vi "Conf EZ.vi"(0 "VISA Resource Name":refnum<visa-resource-name>, 1 "Voltage/Freq/Period Conf":T2={"Range (5:Auto)"=enum."Auto", "Resolution (5:Default)"=enum."Default"}, 2 "Current Conf":T4={"Range (3:Auto)"=enum."Auto", "Resolution (3:Least)"=enum."Least"}, 3 "Resistance Conf":T3={"Range (7:Auto)"=enum."Auto", "Resolution (5:Default)"=enum."Default"}, 5 "Channel List(empty)":string, 7 "Set/Check (F:Set)":bool, 9 "Measurement (1:DC Volt)":T5(ring)=enum."DC Voltage", 11 "error in (no error)":errorcluster, 12 "Temperature Conf":T1={"Transducer Type (0:TC)"=enum."Thermocouple", "Thermocouple Type (8:Last)"=enum."Default (Last)", "Thermistor Type (3: Last)"=enum."Default (Last)", "RTD Type (2:Last)"=enum."Default (Last)"}, 13 "Digital (0:Byte)":u16(ring) items=["Byte"], 14 "Totalizer (0:Read)":enum16{"Read", "Read and Reset"}(ring)) -> (4 "VISA Resource Name Out":refnum<visa-resource-name>, 8 "Configuration?":string, 15 "error out":errorcluster)   [LabVIEW 2018, in "Agilent 34970.lvlib"]
doc: "This VI lets you configure the instrument for simple voltage, current, resistance, temperature, freq/period and, digital/totalizer measurements as well as setting up the scan list. Looking at the block diagram of \"HP34970A Advanced Scan Example.vi\", this VI replaces the specific measurment configuration commands (e.g. Conf Voltage) as well as the Conf Scan List VI. The trigger and read VIs are still needed to take a measurement. For more information on the different ways to take a measurment, refer to the context help and block diagram of the \"HP34970A Advanced Scan Example.vi\".\n\n* Note * There was a bug in the old driver giving the option to read a word from the digital port. This is not possible with the CONF command. To read a word, according to the documentation, put both digital input channels in the same scan list. The readings will be taken simultaneously and given the same timestamp."
uses:
  Agilent 34970.lvlib
panel:
  out "Command":string
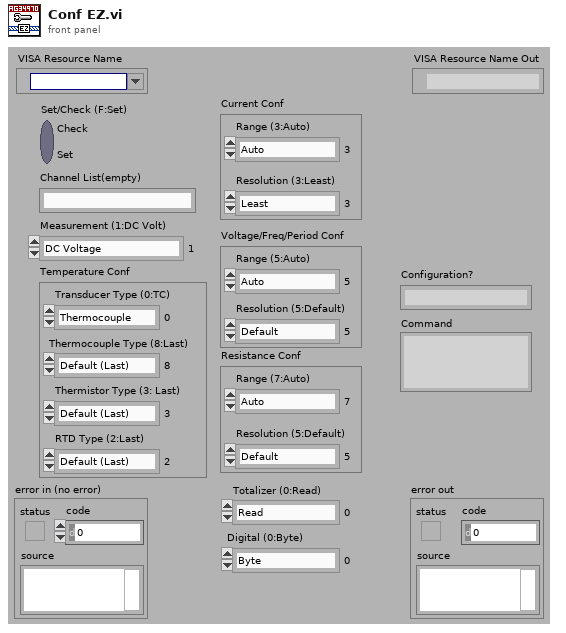
[diagram p1: front panel]
types:
  T1 = cluster{"Transducer Type (0:TC)":enum16{"Thermocouple", "Thermistor", "RTD", "4-Wire RTD", "Default (Last)"}, "Thermocouple Type (8:Last)":enum16{"B", "E", "J", "K", "N", "R", "S", "T", "Default (Last)"}, "Thermistor Type (3: Last)":enum16{"2252", "5000", "10000", "Default (Last)"}, "RTD Type (2:Last)":enum16{"85", "91", "Default (Last)"}}
  T2 = cluster{"Range (5:Auto)":enum16{"100 mV", "1 V", "10 V", "100 V", "300 V", "Auto", "Minimum", "Maximum"}, "Resolution (5:Default)":enum16{"4 1/2", "5 1/2", "6 1/2", "Least", "Highest", "Default"}}
  T3 = cluster{"Range (7:Auto)":enum16{"100 Ohm", "1 kOhm", "10 kOhm", "100 kOhm", "1 MOhm", "10 MOhm", "100 MOhm", "Auto", "Minimum", "Maximum"}, "Resolution (5:Default)":enum16{"4 1/2", "5 1/2", "6 1/2", "Least", "Highest", "Default"}}
  T4 = cluster{"Range (3:Auto)":enum16{"10 mA", "100 mA", "1 A", "Auto", "Minimum", "Maximum"}, "Resolution (3:Least)":enum16{"4 1/2", "5 1/2", "6 1/2", "Least", "Highest", "Default"}}
  T5 = enum16{"Temperature", "DC Voltage", "AC Voltage", "DC Current", "AC Current", "Resistance", "4-Wire Resistance", "Frequency", "Period", "Digital", "Totalizer"}
  T6 = enum16{"Thermocouple", "Thermistor", "RTD", "4-Wire RTD", "Default (Last)"}
  T7 = enum16{"B", "E", "J", "K", "N", "R", "S", "T", "Default (Last)"}
  T8 = enum16{"2252", "5000", "10000", "Default (Last)"}
  T9 = enum16{"100 mV", "1 V", "10 V", "100 V", "300 V", "Auto", "Minimum", "Maximum"}
  T10 = enum16{"4 1/2", "5 1/2", "6 1/2", "Least", "Highest", "Default"}
  T11 = enum16{"100 Ohm", "1 kOhm", "10 kOhm", "100 kOhm", "1 MOhm", "10 MOhm", "100 MOhm", "Auto", "Minimum", "Maximum"}
  T12 = enum16{"10 mA", "100 mA", "1 A", "Auto", "Minimum", "Maximum"}
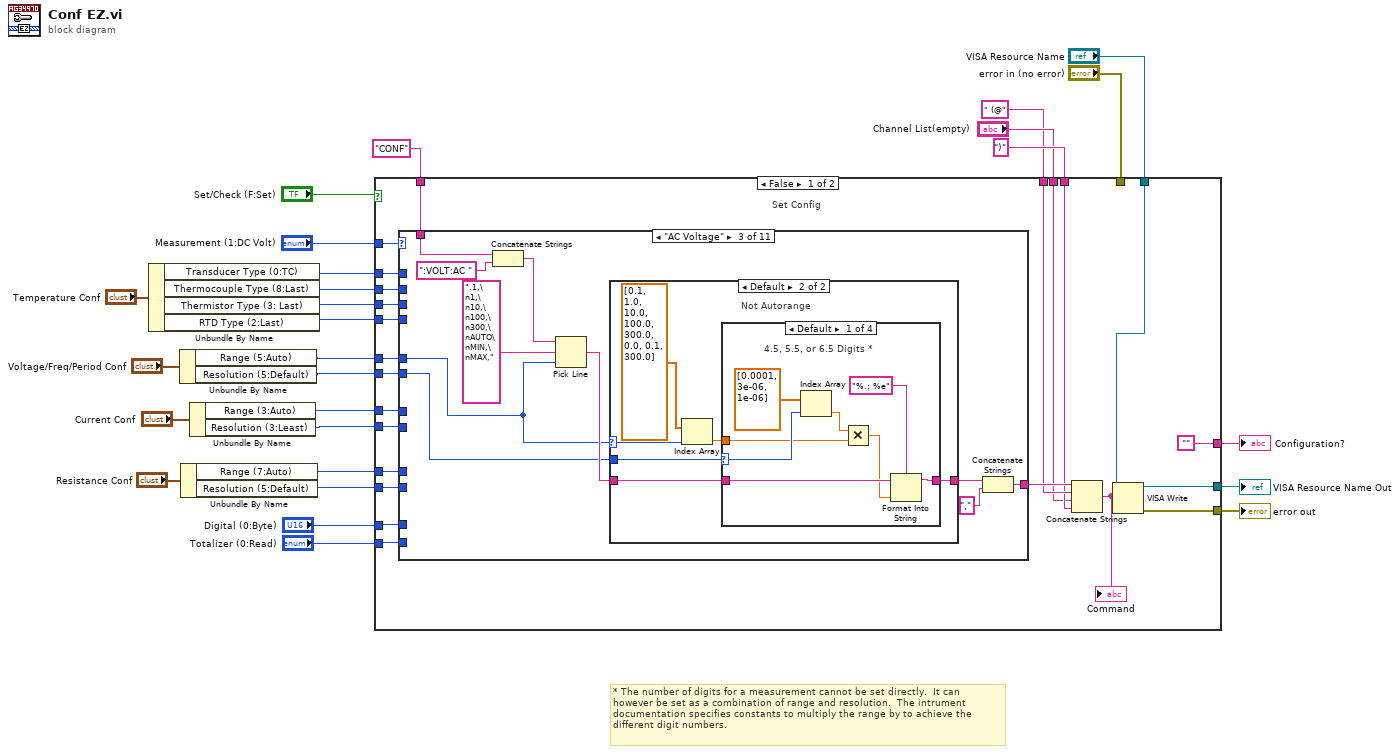
[diagram p0: block diagram]
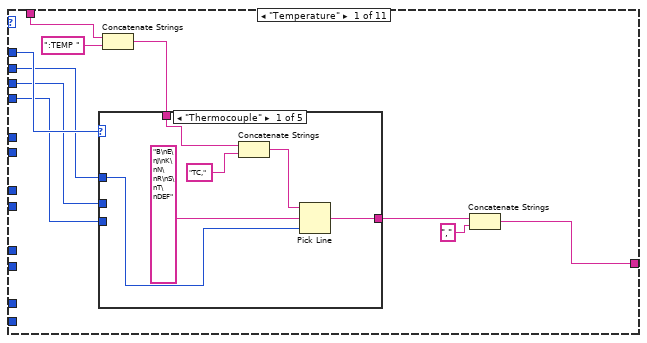
[diagram p2: hidden frame]
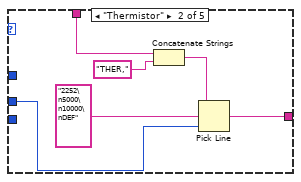
[diagram p3: hidden frame]
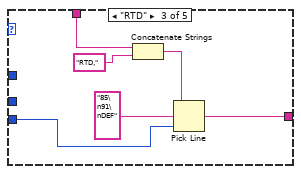
[diagram p4: hidden frame]
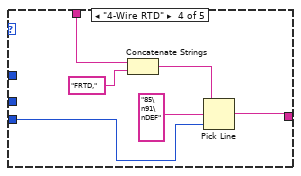
[diagram p5: hidden frame]
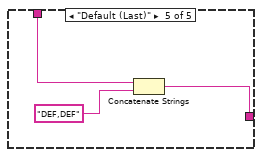
[diagram p6: hidden frame]
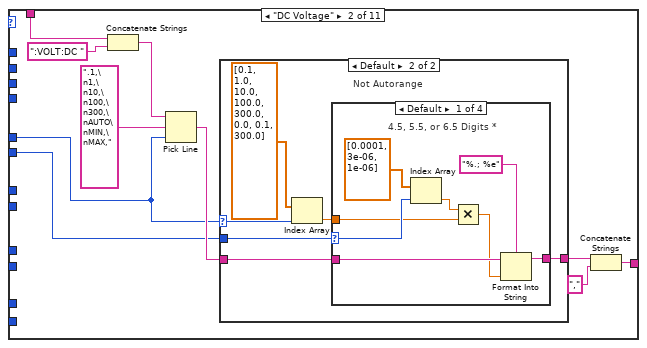
[diagram p7: hidden frame]
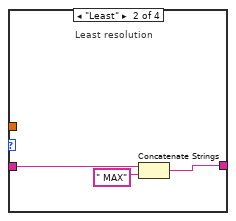
[diagram p9: hidden frame]
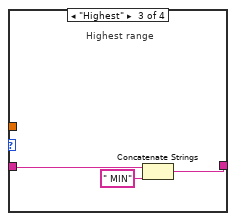
[diagram p10: hidden frame]
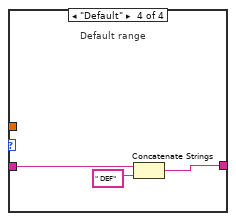
[diagram p11: hidden frame]
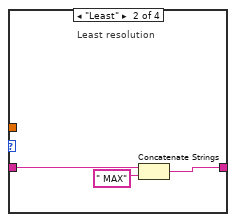
[diagram p13: hidden frame]
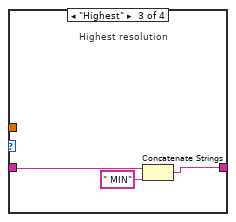
[diagram p14: hidden frame]
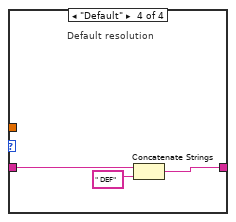
[diagram p15: hidden frame]
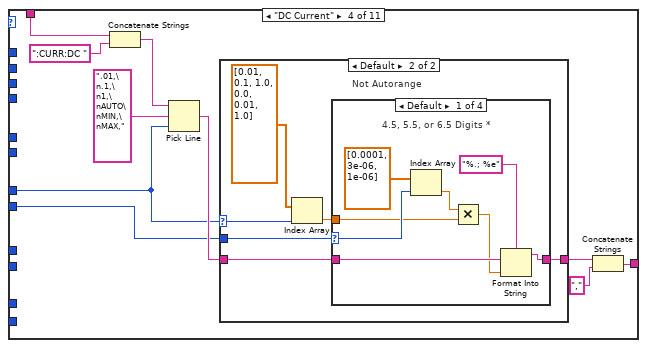
[diagram p16: hidden frame]
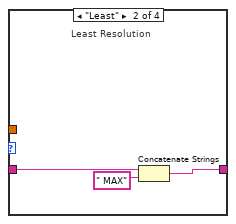
[diagram p18: hidden frame]
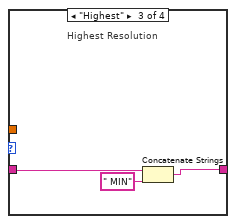
[diagram p19: hidden frame]
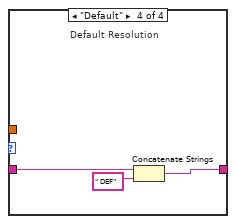
[diagram p20: hidden frame]
diagram:
  # "* The number of digits for a measurement cannot be set directly.  It can\nhowever be set as a combination of range and resolution.  The intrument\ndocumentation specifies constants to multiply the range by to achieve the\ndifferent digit numbers."
  n1 = Unbundle By Name("Temperature Conf") -> ("Transducer Type (0:TC)"=w17:T6, "Thermocouple Type (8:Last)"=w16:T7, "Thermistor Type (3: Last)"=w15:T8, "RTD Type (2:Last)"=w14:enum16{"85", "91", "Default (Last)"})
  n2 = Unbundle By Name("Voltage/Freq/Period Conf") -> ("Range (5:Auto)"=w12:T9, "Resolution (5:Default)"=w11:T10)
  n3 = Unbundle By Name("Resistance Conf") -> ("Range (7:Auto)"=w6:T11, "Resolution (5:Default)"=w5:T10)
  n4 = Unbundle By Name("Current Conf") -> ("Range (3:Auto)"=w9:T12, "Resolution (3:Least)"=w8:T10)
  n5 = case shown="False" "Set/Check (F:Set)" {
    tunnel: " (@" -> [w34 w313]
    tunnel: "Channel List(empty)" -> [w31 w326]
    tunnel: ")" -> [w33 w325]
    tunnel: "Totalizer (0:Read)" -> [w50 _]
    tunnel: "Digital (0:Byte)" -> [w49 _]
    tunnel: w14 -> [w48 _]
    tunnel: w15 -> [w47 _]
    tunnel: w16 -> [w46 _]
    tunnel: w17 -> [w45 _]
    tunnel: "Measurement (1:DC Volt)" -> [w44 _]
    tunnel: "CONF" -> [w43 w324]
    tunnel: "VISA Resource Name" -> [w30 w322]
    tunnel: "error in (no error)" -> [_ w321]
    tunnel: ["" w317] -> w19
    tunnel: [w28 w316] -> w4
    tunnel: [w29 w315] -> w3
    tunnel: w12 -> [w41 _]
    tunnel: w11 -> [w40 _]
    tunnel: w9 -> [w39 _]
    tunnel: w8 -> [w38 _]
    tunnel: w6 -> [w37 _]
    tunnel: w5 -> [w36 _]
    frame False {
      # "Set Config"
      n6 = case shown="\"AC Voltage\"" w44 {
        tunnel: w45 -> [w58 _ _ _ _ _ _ _ _ _ _]
        tunnel: w46 -> [w57 _ _ _ _ _ _ _ _ _ _]
        tunnel: w47 -> [w56 _ _ _ _ _ _ _ _ _ _]
        tunnel: w48 -> [w55 _ _ _ _ _ _ _ _ _ _]
        tunnel: w43 -> [w54 w96 w130 w164 w198 w232 w266 w296 w302 w306 w310]
        tunnel: w49 -> [_ _ _ _ _ _ _ _ _ _ _]
        tunnel: w50 -> [_ _ _ _ _ _ _ _ _ _ w311]
        tunnel: w41 -> [_ w91 w125 _ _ _ _ w293 w298 _ _]
        tunnel: w40 -> [_ w92 w126 _ _ _ _ _ _ _ _]
        tunnel: w39 -> [_ _ _ w160 w194 _ _ _ _ _ _]
        tunnel: w38 -> [_ _ _ w159 w193 _ _ _ _ _ _]
        tunnel: w37 -> [_ _ _ _ _ w228 w262 _ _ _ _]
        tunnel: w36 -> [_ _ _ _ _ w227 w261 _ _ _ _]
        tunnel: [w52 w89 w122 w157 w191 w225 w258 w292 w299 w305 w307] -> w35
        frame "Temperature" {
          n7 = Concatenate Strings(w54, ":TEMP ") -> (w59:string)
          n8 = case shown="\"Thermocouple\"" w58 {
            tunnel: w59 -> [w65 w68 w75 w80 w86]
            tunnel: [w62 w69 w74 w81 w85] -> w53
            tunnel: w57 -> [w61 _ _ _ _]
            tunnel: w56 -> [_ w67 _ _ _]
            tunnel: w55 -> [_ _ w73 w79 _]
            frame "Thermocouple" {
              n9 = Concatenate Strings(w65, "TC,") -> (w63:string)
              n10 = Pick Line(string ("")=w63, multi-line string="B\nE\nJ\nK\nN\nR\nS\nT\nDEF", line index=w61) -> (output string=w62:string)
            }
            frame "Thermistor" {
              n11 = Concatenate Strings(w68, "THER,") -> (w70:string)
              n12 = Pick Line(string ("")=w70, multi-line string="2252\n5000\n10000\nDEF", line index=w67) -> (output string=w69:string)
            }
            frame "RTD" {
              n13 = Concatenate Strings(w75, "RTD,") -> (w78:string)
              n14 = Pick Line(string ("")=w78, multi-line string="85\n91\nDEF", line index=w73) -> (output string=w74:string)
            }
            frame "4-Wire RTD" {
              n15 = Concatenate Strings(w80, "FRTD,") -> (w84:string)
              n16 = Pick Line(string ("")=w84, multi-line string="85\n91\nDEF", line index=w79) -> (output string=w81:string)
            }
            frame "Default (Last)" {
              n17 = Concatenate Strings(w86, "DEF,DEF") -> (w85:string)
            }
          }
          n18 = Concatenate Strings(w53, "," ("string")) -> (w52:string)
        }
        frame "DC Voltage" {
          n19 = Concatenate Strings(w96, ":VOLT:DC ") -> (w94:string)
          n20 = Pick Line(string ("")=w94, multi-line string=".1,\n1,\n10,\n100,\n300,\nAUTO\nMIN,\nMAX,", line index=w91) -> (output string=w93:string)
          n21 = case shown="Default" w91 {
            selector: w91 -> [_ w104]
            tunnel: [w98 w101] -> w90
            tunnel: w93 -> [w98 w100]
            tunnel: w92 -> [_ w102]
            frame "Auto" {
              # "Autorange"
            }
            frame Default {
              # "Not Autorange"
              n22 = Index Array(array=dbl[] [0.1, 1.0, 10.0, 100.0, 300.0, 0.0, 0.1, 300.0], index=w104) -> (element=w99:dbl)
              n23 = case shown="Default" w102 {
                selector: w102 -> [w111 _ _ _]
                tunnel: [w105 w115 w118 w119] -> w101
                tunnel: w100 -> [w108 w114 w116 w120]
                tunnel: w99 -> [w110 _ _ _]
                frame Default {
                  # "4.5, 5.5, or 6.5 Digits *"
                  n24 = Index Array(array=dbl[] [0.0001, 3e-06, 1e-06], index=w111) -> (element=w109:dbl)
                  n25 = Multiply(x=w109, y=w110) -> (x*y=w107:dbl)
                  n26 = Format Into String(format string="%.; %e", initial string=w108, w107) -> (resulting string=w105:string)  [unwired: 1 in, 1 out]
                }
                frame "Least" {
                  # "Least resolution"
                  n27 = Concatenate Strings(w114, " MAX" ("string")) -> (w115:string)
                }
                frame "Highest" {
                  # "Highest range"
                  n28 = Concatenate Strings(w116, " MIN" ("string")) -> (w118:string)
                }
                frame "Default" {
                  # "Default range"
                  n29 = Concatenate Strings(w120, " DEF" ("string")) -> (w119:string)
                }
              }
            }
          }
          n30 = Concatenate Strings(w90, "," ("string")) -> (w89:string)
        }
        frame "AC Voltage" {
          n31 = Concatenate Strings(w130, ":VOLT:AC ") -> (w128:string)
          n32 = Pick Line(string ("")=w128, multi-line string=".1,\n1,\n10,\n100,\n300,\nAUTO\nMIN,\nMAX,", line index=w125) -> (output string=w127:string)
          n33 = case shown="Default" w125 {
            selector: w125 -> [_ w138]
            tunnel: [w132 w135] -> w123
            tunnel: w127 -> [w132 w134]
            tunnel: w126 -> [_ w136]
            frame "Auto" {
              # "Autorange"
            }
            frame Default {
              # "Not Autorange"
              n34 = Index Array(array=dbl[] [0.1, 1.0, 10.0, 100.0, 300.0, 0.0, 0.1, 300.0], index=w138) -> (element=w133:dbl)
              n35 = case shown="Default" w136 {
                selector: w136 -> [w145 _ _ _]
                tunnel: [w139 w149 w152 w153] -> w135
                tunnel: w134 -> [w142 w148 w150 w154]
                tunnel: w133 -> [w144 _ _ _]
                frame Default {
                  # "4.5, 5.5, or 6.5 Digits *"
                  n36 = Index Array(array=dbl[] [0.0001, 3e-06, 1e-06], index=w145) -> (element=w143:dbl)
                  n37 = Multiply(x=w143, y=w144) -> (x*y=w141:dbl)
                  n38 = Format Into String(format string="%.; %e", initial string=w142, w141) -> (resulting string=w139:string)  [unwired: 1 in, 1 out]
                }
                frame "Least" {
                  # "Least resolution"
                  n39 = Concatenate Strings(w148, " MAX" ("string")) -> (w149:string)
                }
                frame "Highest" {
                  # "Highest resolution"
                  n40 = Concatenate Strings(w150, " MIN" ("string")) -> (w152:string)
                }
                frame "Default" {
                  # "Default resolution"
                  n41 = Concatenate Strings(w154, " DEF" ("string")) -> (w153:string)
                }
              }
            }
          }
          n42 = Concatenate Strings(w123, "," ("string")) -> (w122:string)
        }
        frame "DC Current" {
          n43 = Concatenate Strings(w164, ":CURR:DC ") -> (w162:string)
          n44 = Pick Line(string ("")=w162, multi-line string=".01,\n.1,\n1,\nAUTO\nMIN,\nMAX,", line index=w160) -> (output string=w161:string)
          n45 = case shown="Default" w160 {
            selector: w160 -> [_ w172]
            tunnel: [w166 w169] -> w156
            tunnel: w161 -> [w166 w168]
            tunnel: w159 -> [_ w170]
            frame "Auto" {
              # "Autorange"
            }
            frame Default {
              # "Not Autorange"
              n46 = Index Array(array=dbl[] [0.01, 0.1, 1.0, 0.0, 0.01, 1.0], index=w172) -> (element=w167:dbl)
              n47 = case shown="Default" w170 {
                selector: w170 -> [w179 _ _ _]
                tunnel: [w173 w183 w186 w187] -> w169
                tunnel: w168 -> [w176 w182 w184 w188]
                tunnel: w167 -> [w178 _ _ _]
                frame Default {
                  # "4.5, 5.5, or 6.5 Digits *"
                  n48 = Index Array(array=dbl[] [0.0001, 3e-06, 1e-06], index=w179) -> (element=w177:dbl)
                  n49 = Multiply(x=w177, y=w178) -> (x*y=w175:dbl)
                  n50 = Format Into String(format string="%.; %e", initial string=w176, w175) -> (resulting string=w173:string)  [unwired: 1 in, 1 out]
                }
                frame "Least" {
                  # "Least Resolution"
                  n51 = Concatenate Strings(w182, " MAX" ("string")) -> (w183:string)
                }
                frame "Highest" {
                  # "Highest Resolution"
                  n52 = Concatenate Strings(w184, " MIN" ("string")) -> (w186:string)
                }
                frame "Default" {
                  # "Default Resolution"
                  n53 = Concatenate Strings(w188, " DEF" ("string")) -> (w187:string)
                }
              }
            }
          }
          n54 = Concatenate Strings(w156, "," ("string")) -> (w157:string)
        }
        frame "AC Current" {
          n55 = Concatenate Strings(w198, ":CURR:AC ") -> (w196:string)
          n56 = Pick Line(string ("")=w196, multi-line string=".01,\n.1,\n1,\nAUTO\nMIN,\nMAX,", line index=w194) -> (output string=w195:string)
          n57 = case shown="Default" w194 {
            selector: w194 -> [_ w206]
            tunnel: [w200 w203] -> w190
            tunnel: w195 -> [w200 w202]
            tunnel: w193 -> [_ w204]
            frame "Auto" {
              # "Autorange"
            }
            frame Default {
              # "Not autorange"
              n58 = Index Array(array=dbl[] [0.01, 0.1, 1.0, 0.0, 0.01, 1.0], index=w206) -> (element=w201:dbl)
              n59 = case shown="\"Least\"" w204 {
                selector: w204 -> [w213 _ _ _]
                tunnel: [w207 w217 w220 w221] -> w203
                tunnel: w202 -> [w210 w216 w218 w222]
                tunnel: w201 -> [w212 _ _ _]
                frame Default {
                  # "4.5, 5.5, or 6.5 Digits *"
                  n60 = Index Array(array=dbl[] [0.0001, 3e-06, 1e-06], index=w213) -> (element=w211:dbl)
                  n61 = Multiply(x=w211, y=w212) -> (x*y=w209:dbl)
                  n62 = Format Into String(format string="%.; %e", initial string=w210, w209) -> (resulting string=w207:string)  [unwired: 1 in, 1 out]
                }
                frame "Least" {
                  # "Least Resolution"
                  n63 = Concatenate Strings(w216, " MAX" ("string")) -> (w217:string)
                }
                frame "Highest" {
                  # "Highest resolution"
                  n64 = Concatenate Strings(w218, " MIN" ("string")) -> (w220:string)
                }
                frame "Default" {
                  # "Default resolution"
                  n65 = Concatenate Strings(w222, " DEF" ("string")) -> (w221:string)
                }
              }
            }
          }
          n66 = Concatenate Strings(w190, "," ("string")) -> (w191:string)
        }
        frame "Resistance" {
          n67 = Concatenate Strings(w232, ":RES ") -> (w230:string)
          n68 = Pick Line(string ("")=w230, multi-line string="1e2,\n1e3,\n10e3,\n100e3,\n1e6,\n10e6,\n100e6,\nAUTO\nMIN,\nMAX,", line index=w228) -> (output string=w229:string)
          n69 = case shown="Default" w228 {
            selector: w228 -> [_ w240]
            tunnel: [w234 w237] -> w224
            tunnel: w229 -> [w234 w236]
            tunnel: w227 -> [_ w238]
            frame "Auto" {
              # "Autorange"
            }
            frame Default {
              # "Not Autorange"
              n70 = Index Array(array=dbl[] [100.0, 1000.0, 10000.0, 100000.0, 1000000.0, 10000000.0, 100000000.0, 0.0, 100.0, 100000000.0], index=w240) -> (element=w235:dbl)
              n71 = case shown="Default" w238 {
                selector: w238 -> [w247 _ _ _]
                tunnel: [w241 w251 w254 w255] -> w237
                tunnel: w236 -> [w244 w250 w252 w256]
                tunnel: w235 -> [w246 _ _ _]
                frame Default {
                  # "4.5, 5.5, or 6.5 Digits *"
                  n72 = Index Array(array=dbl[] [0.0001, 3e-06, 1e-06], index=w247) -> (element=w245:dbl)
                  n73 = Multiply(x=w245, y=w246) -> (x*y=w243:dbl)
                  n74 = Format Into String(format string="%.; %e", initial string=w244, w243) -> (resulting string=w241:string)  [unwired: 1 in, 1 out]
                }
                frame "Least" {
                  # "Least Resolution"
                  n75 = Concatenate Strings(w250, " MAX" ("string")) -> (w251:string)
                }
                frame "Highest" {
                  # "Highest Resolution"
                  n76 = Concatenate Strings(w252, " MIN" ("string")) -> (w254:string)
                }
                frame "Default" {
                  # "Default Resolution"
                  n77 = Concatenate Strings(w256, " DEF" ("string")) -> (w255:string)
                }
              }
            }
          }
          n78 = Concatenate Strings(w224, "," ("string")) -> (w225:string)
        }
        frame "4-Wire Resistance" {
          n79 = Concatenate Strings(w266, ":FRES ") -> (w264:string)
          n80 = Pick Line(string ("")=w264, multi-line string="1e2,\n1e3,\n10e3,\n100e3,\n1e6,\n10e6,\n100e6,\nAUTO\nMIN,\nMAX,", line index=w262) -> (output string=w263:string)
          n81 = case shown="Default" w262 {
            selector: w262 -> [_ w274]
            tunnel: [w268 w271] -> w259
            tunnel: w263 -> [w268 w270]
            tunnel: w261 -> [_ w272]
            frame "Auto" {
              # "Autorange"
            }
            frame Default {
              # "Not Autorange"
              n82 = Index Array(array=dbl[] [100.0, 1000.0, 10000.0, 100000.0, 1000000.0, 10000000.0, 100000000.0, 0.0, 100.0, 100000000.0], index=w274) -> (element=w269:dbl)
              n83 = case shown="Default" w272 {
                selector: w272 -> [w281 _ _ _]
                tunnel: [w275 w285 w288 w289] -> w271
                tunnel: w270 -> [w278 w284 w286 w290]
                tunnel: w269 -> [w280 _ _ _]
                frame Default {
                  # "4.5, 5.5, or 6.5 Digits *"
                  n84 = Index Array(array=dbl[] [0.0001, 3e-06, 1e-06], index=w281) -> (element=w279:dbl)
                  n85 = Multiply(x=w279, y=w280) -> (x*y=w277:dbl)
                  n86 = Format Into String(format string="%.; %e", initial string=w278, w277) -> (resulting string=w275:string)  [unwired: 1 in, 1 out]
                }
                frame "Least" {
                  # "Least Resolution"
                  n87 = Concatenate Strings(w284, " MAX" ("string")) -> (w285:string)
                }
                frame "Highest" {
                  # "Highest Resolution"
                  n88 = Concatenate Strings(w286, " MIN" ("string")) -> (w288:string)
                }
                frame "Default" {
                  # "Default Resolution"
                  n89 = Concatenate Strings(w290, " DEF" ("string")) -> (w289:string)
                }
              }
            }
          }
          n90 = Concatenate Strings(w259, "," ("string")) -> (w258:string)
        }
        frame "Frequency" {
          n91 = Concatenate Strings(w296, ":FREQ 20,") -> (w294:string)
          n92 = Pick Line(string ("")=w294, multi-line string=".1,\n1,\n10,\n100,\n300,\n\nMIN,\nMAX,", line index=w293) -> (output string=w292:string)
        }
        frame "Period" {
          n93 = Concatenate Strings(w302, ":PER .05") -> (w300:string)
          n94 = Pick Line(string ("")=w300, multi-line string=",.1,\n,1,\n,10,\n,100,\n,300,\n,\n,MIN,\n,MAX,", line index=w298) -> (output string=w299:string)
        }
        frame "Digital" {
          # "There was an bug in the old driver giving the option\nto read a word from the digital port.  This is not possible\nwith the CONF command.  To read a word, according to\nthe documentation, put both digital input channels in the\nsame scan list.  The readings will be taken simultaneously \nand given the same timestamp."
          n95 = Concatenate Strings(w306, ":DIG:BYTE " ("string")) -> (w305:string)
        }
        frame "Totalizer" {
          n96 = Pick Line(string ("")=w310, multi-line string=":TOT READ\n:TOT RRES", line index=w311) -> (output string=w309:string)
          n97 = Concatenate Strings(w309, "," ("string")) -> (w307:string)
        }
      }
      n98 = Concatenate Strings(w35, w34, w31, w33) -> (w32:string)
      "Command" <- w32
      n99 = VISA Write(VISA resource name=w30, write buffer=w32) -> (VISA resource name out=w28:refnum<visa-resource-name>, error out=w29:errorcluster)  [unwired: 1 in, 1 out]
    }
    frame True {
      # "Check Config"
      n100 = Concatenate Strings(w324, "? ") -> (w323:string)
      n101 = Concatenate Strings(w323, w313, w326, w325) -> (w314:string)
      n102 = VISA Write(VISA resource name=w322, write buffer=w314, error in (no error)=w321) -> (VISA resource name out=w320:refnum<visa-resource-name>, error out=w319:errorcluster)  [unwired: 1 out]
      n103 = VISA Read(VISA resource name=w320, byte count=u32 100 ("byte count (0)"), error in (no error)=w319) -> (VISA resource name out=w316:refnum<visa-resource-name>, read buffer=w317:string, error out=w315:errorcluster)  [unwired: 1 out]
    }
  }
  "Configuration?" <- w19
  "error out" <- w3
  "VISA Resource Name Out" <- w4
